vi "Raise Navigation Starting Event.vi"(4 "Event in":refnum<user-event>, 5 "Event Data":cluster{"sender":refnum<k24>, "e":refnum<k24>}, 6 "Control Ref":refnum<k24>, 7 "Event Common Data":T1) -> ()   [LabVIEW 2024, in "WebView.lvclass"]
uses:
  WebView.lvclass
  <vilib>/sklein/WebView2/Libs/Microsoft.Web.WebView2.Core.dll
  Navigation Start Event Data--cluster.ctl
  WebView.lvclass/WebView.ctl
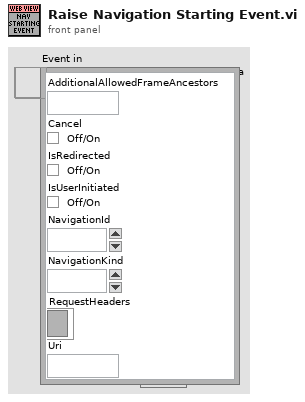
[diagram p1: front panel]
types:
  T1 = cluster{"Event Source":i32, "Event Type":u32, "Time Stamp":u32}
  T2 = typedef "WebView.lvclass/Navigation Start Event Data--cluster.ctl" = cluster{"AdditionalAllowedFrameAncestors":string, "Cancel":bool, "IsRedirected":bool, "IsUserInitiated":bool, "NavigationId":u64, "NavigationKind":i32, "RequestHeaders":refnum<k24>, "Uri":string}
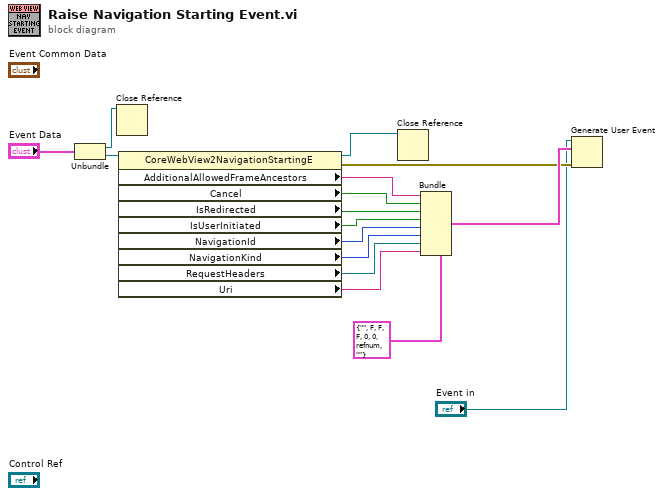
[diagram p0: block diagram]
diagram:
  n1 = Unbundle("Event Data") -> ("sender"=w3:refnum<k24>, "e"=w16:refnum<k24>)
  n2 = Close Reference(reference=w3) -> ()  [unwired: 1 in, 1 out]
  n3 = property class="CoreWebView2NavigationStartingE"(reference=w16) -> (reference out=w2:refnum<k24>, error out=w4:errorcluster, "AdditionalAllowedFrameAncestors"=w14:string, "Cancel"=w13:bool, "IsRedirected"=w12:bool, "IsUserInitiated"=w11:bool, "NavigationId"=w10:u64, "NavigationKind"=w9:i32, "RequestHeaders"=w8:refnum<k24>, "Uri"=w7:string)  [unwired: 1 in]
  n4 = Close Reference(reference=w2) -> ()  [unwired: 1 in, 1 out]
  n5 = Bundle(cluster=T2 {"AdditionalAllowedFrameAncestors"="", "Cancel"=FALSE, "IsRedirected"=FALSE, "IsUserInitiated"=FALSE, "NavigationId"=0, "NavigationKind"=0, "RequestHeaders"=refnum, "Uri"=""} ("Nav Started Event"), "AdditionalAllowedFrameAncestors"=w14, "Cancel"=w13, "IsRedirected"=w12, "IsUserInitiated"=w11, "NavigationId"=w10, "NavigationKind"=w9, "RequestHeaders"=w8, "Uri"=w7) -> (w5:T2)
  n6 = Generate User Event(user event="Event in", event data cluster=w5, error in=w4) -> ()  [unwired: 1 in, 2 out]
